vi "numeric operations.vi"() -> ()   [LabVIEW 2020]
panel:
  out "division":dbl
  out "multiplication":dbl
  out "substraction":dbl
  in  "digit 2":dbl
  out "addition":dbl
  in  "digit 1":dbl
  # "Numeric operations"
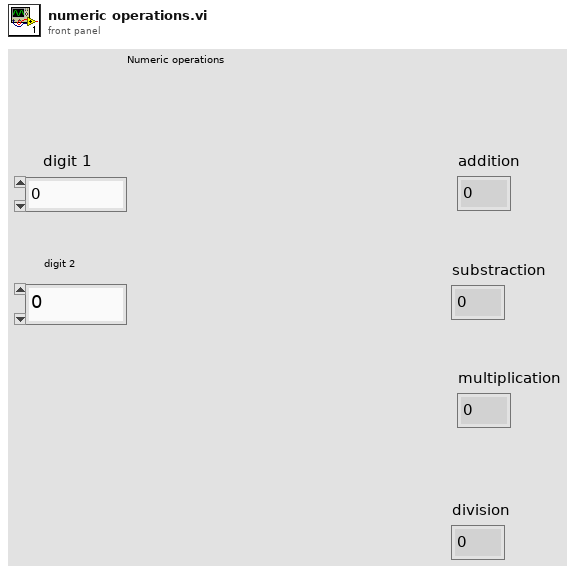
[diagram p1: front panel]
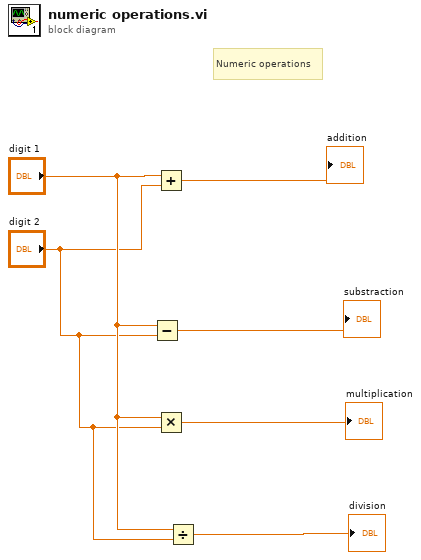
[diagram p0: block diagram]
diagram:
  # "Numeric operations"
  n1 = Subtract(x="digit 1", y="digit 2") -> (x-y=→"substraction":dbl)
  n2 = Add(x="digit 1", y="digit 2") -> (x+y=→"addition":dbl)
  n3 = Multiply(x="digit 1", y="digit 2") -> (x*y=→"multiplication":dbl)
  n4 = Divide(x="digit 1", y="digit 2") -> (x/y=→"division":dbl)
